vi "placeholder--create.vi"(11 "TEMPLATE Actor in":refnum<class "TEMPLATE Actor.lvclass">) -> (0 "Error out":errorcluster, 3 "TEMPLATE Actor out":refnum<class "TEMPLATE Actor.lvclass">)   [LabVIEW 2025, in "_Template.lvlib" / "Templates.lvlib" / "TEMPLATE Actor.lvlib" / "TEMPLATE Actor.lvclass"]
uses:
  TEMPLATE Actor.lvclass
  TEMPLATE Actor.lvclass/TEMPLATE Actor.ctl
  C:/git/jettl/src/jettl Tools/_Template/Templates/TEMPLATE Actor/TEMPLATE Actor/TEMPLATE Actor.lvclass
  C:/git/jettl/src/jettl/jettl/Actor/Actor/Actor.lvclass
  C:/git/jettl/src/jettl/jettl/Terminated Msg/Terminated/Terminated.lvclass
  jettl/jettl/Actor/Actor.lvlib
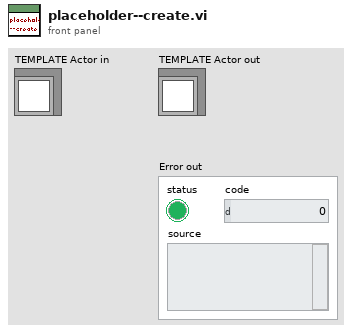
[diagram p1: front panel]
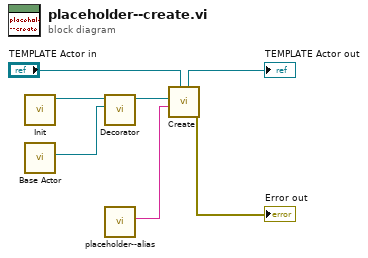
[diagram p0: block diagram]
diagram:
  n1 = call "Init.vi"() -> ("TEMPLATE Actor out"=w7:refnum<class "TEMPLATE Actor.lvclass">)  [unwired: 11 in]
  n2 = call "Base Actor.vi"() -> ("Actor"=w6:refnum<class "Actor.lvclass">)  [unwired: 11 in]
  n3 = call-dynamic "Decorator.vi"("Actor"=w6, "TEMPLATE Actor in"=w7) -> ("TEMPLATE Actor out"=w2:refnum<class "TEMPLATE Actor.lvclass">)  [unwired: 9 in]
  n4 = call "placeholder--alias.vi"() -> ("Prefix"=w1:string)  [unwired: 11 in]
  n5 = call "Create.vi"("Actor in"="TEMPLATE Actor in", "Alias"=w1, "Actor"=w2) -> ("Error out"=→"Error out":errorcluster, "Actor out"=→"TEMPLATE Actor out":refnum<class "TEMPLATE Actor.lvclass">)  [unwired: 7 in]
